vi "Simple UDP - Receiver.vi"() -> ()   [LabVIEW 2017]
doc: "The UDP protocol differs from TCP in that there is no error-checking with the packets of information that are sent, and thus no guarantee whatsoever that an intended recipient will actually receive a given piece of data.\n\nUDP does offer the ability to \"broadcast\" data across a network--simply specify an IP Address of all ones (255.255.255.255) to attempt to broadcast information network-wide. Keep in mind that routers and other network hardware will generally refuse to forward the broadcast beyond certain points, so the extent of the broadcast will in practice be limited."
panel:
  out "rest of the binary string":string
  out "data out":string
  out "Received Data":dbl(graph)
  in  "Stop":bool
  # "Overview: Demonstrates the use of the UDP functions to receive data over a UDP connection.\nInstructions:\n1. Ensure Simple UDP - Sender.vi is already running.\n2. Run the VI.\n3. Click Stop to stop the VI."
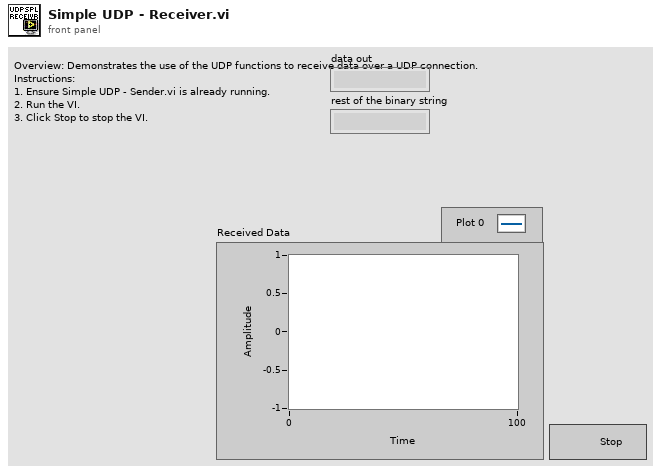
[diagram p1: front panel]
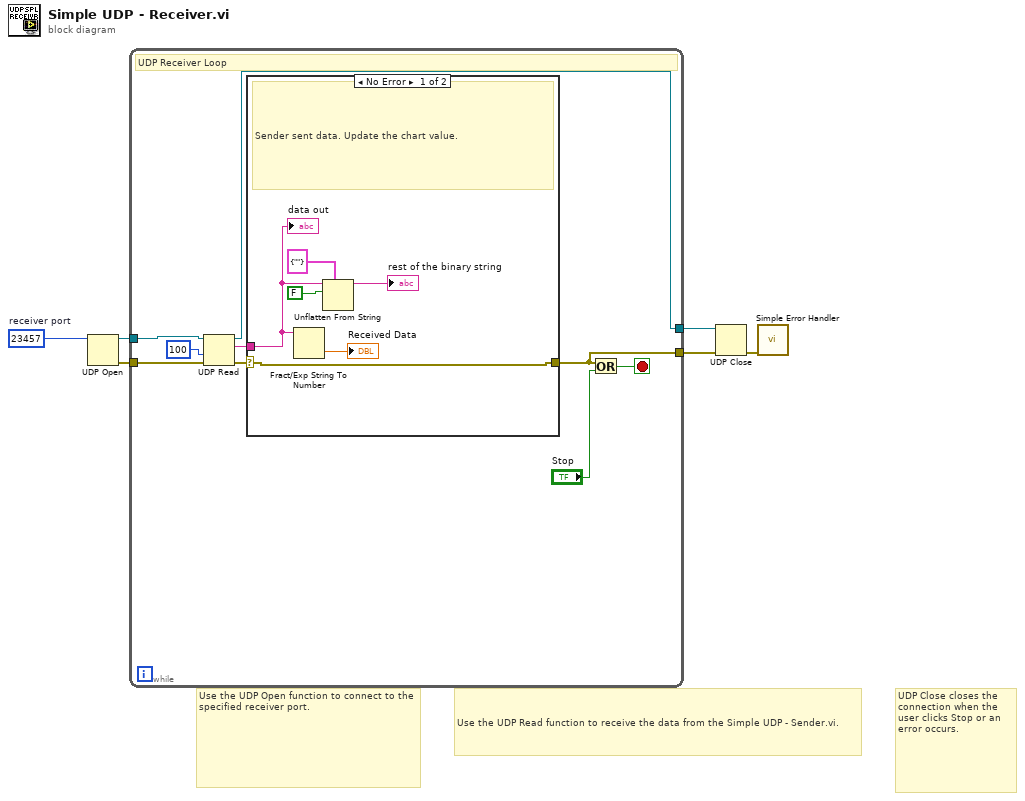
[diagram p0: block diagram]
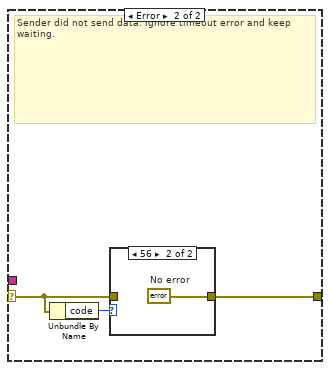
[diagram p2: hidden frame]
diagram:
  w1 = u16 23457  # receiver port
  # "UDP Close closes the connection when the user clicks Stop or an error occurs."
  # "Use the UDP Open function to connect to the specified receiver port."
  # "Use the UDP Read function to receive the data from the Simple UDP - Sender.vi."
  n1 = UDP Open(11:w1) -> (port=w2:refnum<k16>, 0:w3:errorcluster)  [unwired: 4 in, 1 out]
  n2 = while {
    tunnel: w2 -> [w15]
    tunnel: [w7] -> w6
    tunnel: w3 -> [w12]
    tunnel: [w8] -> w4
    stop <- w13 stop-if-true
    # "UDP Receiver Loop"
    n3 = UDP Read(connection ID=w15, timeout ms (25000)=100, 8:w12) -> (data out=w10:string, error out=w9:errorcluster, 3:w7:refnum<k16>)  [unwired: 3 out]
    n4 = case shown="No Error" w9 {
      selector: w9 -> [w20 w23]
      tunnel: w10 -> [w18 _]
      tunnel: [w20 w22] -> w8
      frame No Error {
        # "Sender sent data. Update the chart value."
        n5 = Fract/Exp String To Number(string=w18) -> (number=→"Received Data":dbl)  [unwired: 3 in, 1 out]
        n6 = Unflatten From String(type=cluster{string} {""}, binary string=w18, data includes array or string size? (T)=FALSE) -> (rest of the binary string=→"rest of the binary string":string)  [unwired: 2 in, 2 out]
        "data out" <- w18
      }
      frame Error {
        # "Sender did not send data. Ignore timeout error and keep waiting."
        n7 = Unbundle By Name(w23) -> ("code"=w24:i32)
        n8 = case shown="56" w24 {
          tunnel: w23 -> [w25 _]
          tunnel: [w25 w26] -> w22
          frame Default {
          }
          frame 56 {
            w26 = errorcluster {"status"=FALSE, "code"=0, "source"=""}  # No error
          }
        }
      }
    }
    n9 = Or(x=w8, y="Stop") -> (x .or. y?=w13:bool)
  }
  n10 = UDP Close(connection ID=w6, 8:w4) -> (error out=w5:errorcluster)  [unwired: 1 out]
  n11 = call <vilib>:"Simple Error Handler.vi"("error in (no error)"=w5) -> ()  [unwired: 1 in, 8 out]
